vi "Buffer Packet and Count Size.vi"(0 "serialized data in":u8[](array[numeric])=[0, 0, 0, 0, 0, 0, 0, 0], 1 "reset":bool, 5 "valid bytes in":fxp<+,4,4>, 7 "end of packet":bool, 9 "input valid":bool, 12 "ready for output":bool) -> (4 "serialized data out":u8[](array[numeric]), 6 "valid bytes out":fxp<+,4,4>, 8 "empty":bool, 10 "output valid":bool, 14 "ready for input":bool, 15 "in reset":bool)   [LabVIEW 2020, in "GettingStarted_Acq_Tap_148X_FPGA.lvlib"]
uses:
  GettingStarted_Acq_Tap_148X_FPGA.lvlib
  <vilib>/rvi/DataTransferAndStorage/Container/Common/niFpgaContainerGetUniqueNameForEmu.vi
  <vilib>/rvi/DataTransferAndStorage/Container/Common/niFpgaContainerSetEmuInfo.vi
  <vilib>/rvi/eio/common/nirviEmuReportErrorAndStop.vi
  <vilib>/rvi/LocalResourceManager/LocalResourceManager.xnode
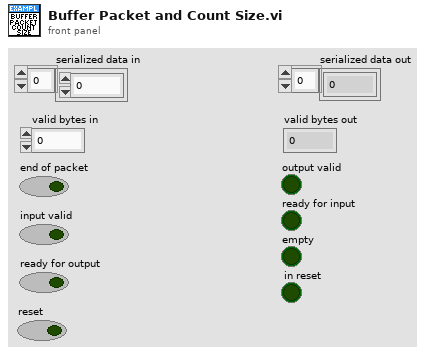
[diagram p1: front panel]
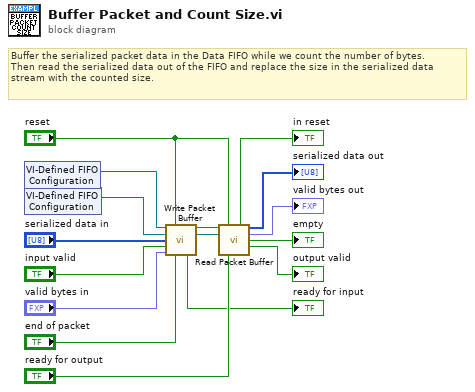
[diagram p0: block diagram]
diagram:
  # "Buffer the serialized packet data in the Data FIFO while we count the number of bytes.\nThen read the serialized data out of the FIFO and replace the size in the serialized data stream with the counted size."
  n1 = xnode "VI-Defined FIFO Configuration"() -> ("FIFO Out"=w4:refnum<k21>)
  n2 = xnode "VI-Defined FIFO Configuration"() -> ("FIFO Out"=w14:refnum<k21>)
  n3 = call "Write Packet Buffer.vi"("data fifo in"=w4, "reset"="reset", "sizes fifo in"=w14, "serialized data"="serialized data in", "input valid"="input valid", "valid bytes in"="valid bytes in", "end of packet"="end of packet") -> ("data fifo out"=w3:refnum<k21>, "sizes fifo out"=w11:refnum<k21>, "ready for input"=→"ready for input":bool)  [unwired: 6 in]
  n4 = call "Read Packet Buffer.vi"("data fifo"=w3, "reset"="reset", "sizes fifo"=w11, "ready for output"="ready for output") -> ("in reset"=→"in reset":bool, "serialized data"=→"serialized data out":u8[], "valid bytes"=→"valid bytes out":fxp<+,4,4>, "empty"=→"empty":bool, "output valid"=→"output valid":bool)  [unwired: 7 in]
